vi "writeToXML.vi"(8 "error in (no error)":errorcluster, 10 "Class Label":string, 11 "Wrapnum in":refnum<class "Wrapnum.lvclass">) -> (0 "error out":errorcluster, 2 "XML out":string, 3 "Wrapnum out":refnum<class "Wrapnum.lvclass">)   [LabVIEW 2010, in "TCS.lvlib" / "TCSDataDefinitions.lvlib" / "TCSCommand.lvlib" / "Wrapnum.lvclass"]
uses:
  Wrapnum.lvclass
  Wrapnum.lvclass/Wrapnum.ctl
  Common/XML/XML.lvlib
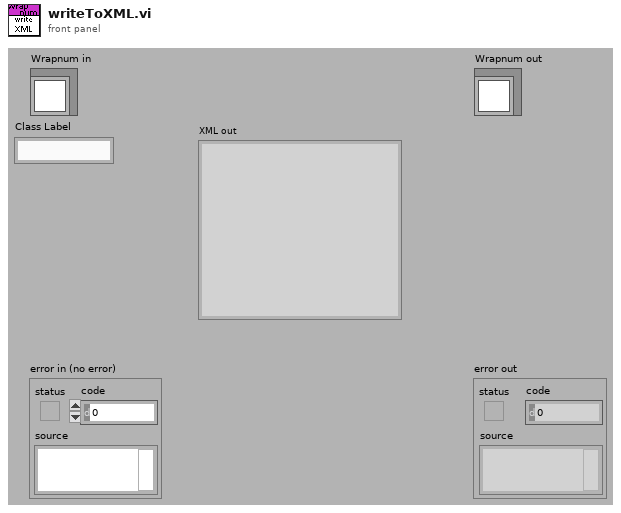
[diagram p1: front panel]
types:
  T1 = typedef "TCS.lvlib/TCSDataDefinitions.lvlib/TCSCommand.lvlib/WrapnumTypes.ctl" = enum16{"-1", "0", "1"}
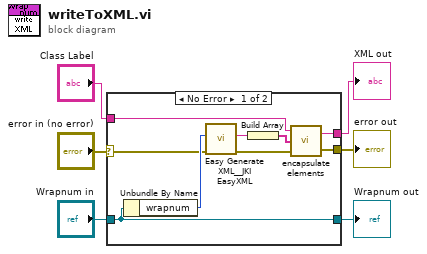
[diagram p0: block diagram]
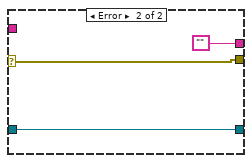
[diagram p2: hidden frame]
diagram:
  n1 = case shown="No Error" "error in (no error)" {
    selector: "error in (no error)" -> [w13 w18]
    tunnel: [w8 w18] -> w5
    tunnel: [w14 w17] -> w3
    tunnel: "Wrapnum in" -> [w14 w17]
    tunnel: "Class Label" -> [w10 _]
    tunnel: [w9 ""] -> w1
    frame No Error {
      n2 = Unbundle By Name(w14) -> ("wrapnum"=w15:T1)
      n3 = call <vilib>:"Easy Generate XML__JKI EasyXML.vi"("error in (no error)"=w13, "LabVIEW Data"=w15) -> ("error out"=w7:errorcluster, "XML String"=w12:string)  [unwired: 8 out]
      n4 = Build Array(w12) -> (w11:string[])
      n5 = call "encapsulate elements.vi"("error in"=w7, "Elements"=w11, "Class Label"=w10) -> ("error out"=w8:errorcluster, "XML out"=w9:string)
    }
    frame Error {
    }
  }
  "error out" <- w5
  "Wrapnum out" <- w3
  "XML out" <- w1
